vi "DataReceived.vi"(8 "error in (no error)":errorcluster, 9 "TimeStamp":timestamp, 10 "Data":string, 11 "Refnum":u64) -> (0 "error out":errorcluster, 3 "DataReceived":refnum<class "DataReceived.lvclass">)   [LabVIEW 2022 SP3, in "Tcp.lvlib" / "DataReceived.lvclass"]
uses:
  DataReceived.lvclass
  DataReceived.lvclass/DataReceived.ctl
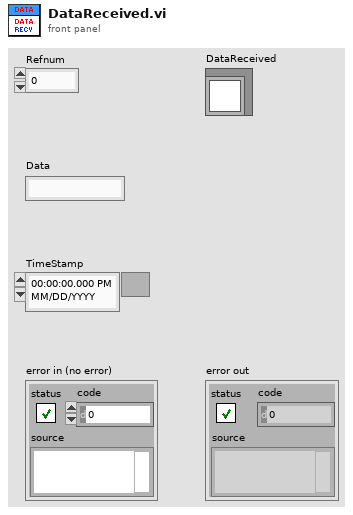
[diagram p1: front panel]
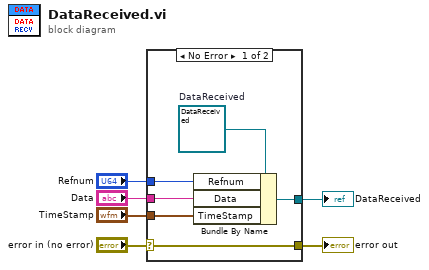
[diagram p0: block diagram]
diagram:
  n1 = case shown="No Error" "error in (no error)" {
    selector: "error in (no error)" -> [w12 w13]
    tunnel: [w12 w13] -> w5
    tunnel: "Refnum" -> [w10 _]
    tunnel: "TimeStamp" -> [w8 _]
    tunnel: "Data" -> [w9 _]
    tunnel: [w7 _] -> w1
    frame No Error {
      w11 = refnum<class "DataReceived.lvclass"> refnum  # DataReceived
      n2 = Bundle By Name(cluster=w11, "Refnum"=w10, "Data"=w9, "TimeStamp"=w8) -> (w7:refnum<class "DataReceived.lvclass">)
    }
    frame Error {
    }
  }
  "error out" <- w5
  "DataReceived" <- w1
